vi "Actor Core.vi"(8 "error in":errorcluster, 11 "Arduino_Stepper in":refnum<class "Arduino_Stepper_UI.lvclass">) -> (0 "error out":errorcluster, 3 "Actor out":refnum<class "Actor.lvclass">)   [LabVIEW 2023, in "Arduino_TranslationStage_UI.lvlib" / "Arduino_Stepper_UI.lvclass"]
doc: "(<B>Filename</B>: Actor Framework.lvlib:Actor.lvclass:Actor Core.vi)\n\nReceives messages to the actor, reacts to them, and initiates any error handling that may shut the actor down.\n\nDescendant classes may override this VI to append parallel tasks for the actor to complete while it handles messages. Overrides use the Call Parent Class Method node."
uses:
  Arduino_Stepper_UI.lvclass
  C:/Program Files/National Instruments/LabVIEW 2023/vi.lib/ActorFramework/Actor/Actor.lvclass
  <vilib>/ActorFramework/Actor/Actor.lvclass
  <vilib>/ActorFramework/Message Enqueuer/Message Enqueuer.lvclass
  ConcreteClasses/ConcreteInstrumentClasses/Arduino_Stepper/Arduino_Stepper/ArduinoTranslationStage.lvclass
  <vilib>/ActorFramework/Actor/Actor.lvclass/Actor.ctl
  <vilib>/ActorFramework/Message Enqueuer/Message Enqueuer.lvclass/Message Enqueuer.ctl
  Arduino_Stepper_UI.lvclass/Arduino_Stepper_UI.ctl
  Top_Controllers/Spectroscopy_Controller/Camera_Scan_Controller Messages/Control_Init_Done Msg/Control_Init_Done Msg.lvclass/Control_Init_Done Msg.ctl
  Interfaces/InitDeinitInterface/InitDeinit Messages/Init Msg/Init Msg.lvclass/Init Msg.ctl
  Interfaces/AbstractInstrumentClasses/TranslationStages_LV/TranslationStagesInterface Messages/MoveBySteps Msg/MoveBySteps Msg.lvclass/MoveBySteps Msg.ctl
  Top_Controllers/Spectroscopy_Controller/Camera_Scan_Controller Messages/InitScan Msg/InitScan Msg.lvclass/InitScan Msg.ctl
  <vilib>/ActorFramework/Message Enqueuer/Init from Existing Queue.vi
  <vilib>/ActorFramework/Message Enqueuer/Enqueue.vi
  Top_Controllers/Spectroscopy_Controller/Camera_Scan_Controller Messages/Control_Init_Done Msg/Control_Init_Done Msg.lvclass
  C:/Program Files/National Instruments/LabVIEW 2023/vi.lib/ActorFramework/Message/Message.lvclass
  Interfaces/InitDeinitInterface/InitDeinit Messages/Init Msg/Init Msg.lvclass
  <vilib>/ActorFramework/Stop Msg/Stop Msg.lvclass
  Top_Controllers/Spectroscopy_Controller/Camera_Scan_Controller Messages/Control_DeInit_Done Msg/Control_DeInit_Done Msg.lvclass
  Interfaces/AbstractInstrumentClasses/TranslationStages_LV/TranslationStagesInterface Messages/MoveBySteps Msg/MoveBySteps Msg.lvclass
  Top_Controllers/Spectroscopy_Controller/Camera_Scan_Controller Messages/InitScan Msg/InitScan Msg.lvclass
  Top_Controllers/Spectroscopy_Controller/Camera_Scan_Controller Messages/Control_Moved Msg/Control_Moved Msg.lvclass
  <vilib>/ActorFramework/Message Priority Queue/Priority Enqueue.vi
panel:
  in  "Delay (ms)":u16(slide) max=5000 step=100 scale=0.0..5000.0
  out "Front Panel":refnum<vi>
  out "Is Top Actor":bool
  out "Caller Enqueuer":refnum<class "Message Enqueuer.lvclass">
  out "Direction":enum16{"Forward", "Backwards"}(ring)
  out "Scanning":bool=TRUE
  out "Moving":bool=TRUE
  out "Exited":bool=TRUE
  out "Connected":bool=TRUE
  out "Self Enqueuer":refnum<class "Message Enqueuer.lvclass">
  out "Arduino Enqueuer":refnum<class "Message Enqueuer.lvclass">
  out "VI":refnum<vi>
  in  "Get Images":bool
  in  "Scan Backwards":bool
  in  "Scan Forward":bool
  in  "Connect":bool
  in  "VISA resource name":refnum<visa-resource-name>
  in  "Jog Backwards":bool
  in  "Jog Forward":bool
  in  "Segments":dbl(slide) min=0.0 max=1000.0 step=1.0 scale=0.0..1000.0
  in  "Speed":dbl(slide)=100.0 min=100.0 max=2000.0 step=1.0 scale=100.0..2000.0
  in  "Steps":dbl(slide)=1.0 min=1.0 max=100000.0 step=1.0 scale=1.0..100000.0
  in  "Stop Button":bool
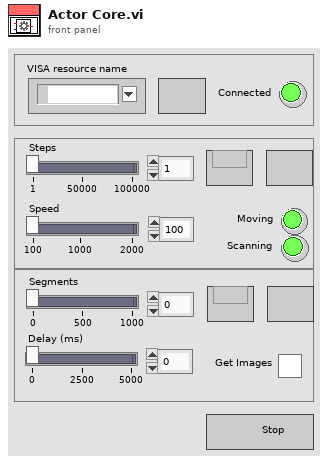
[diagram p1: front panel]
types:
  T1 = enum8{"Enabled", "Disabled", "Disabled and Grayed Out"}
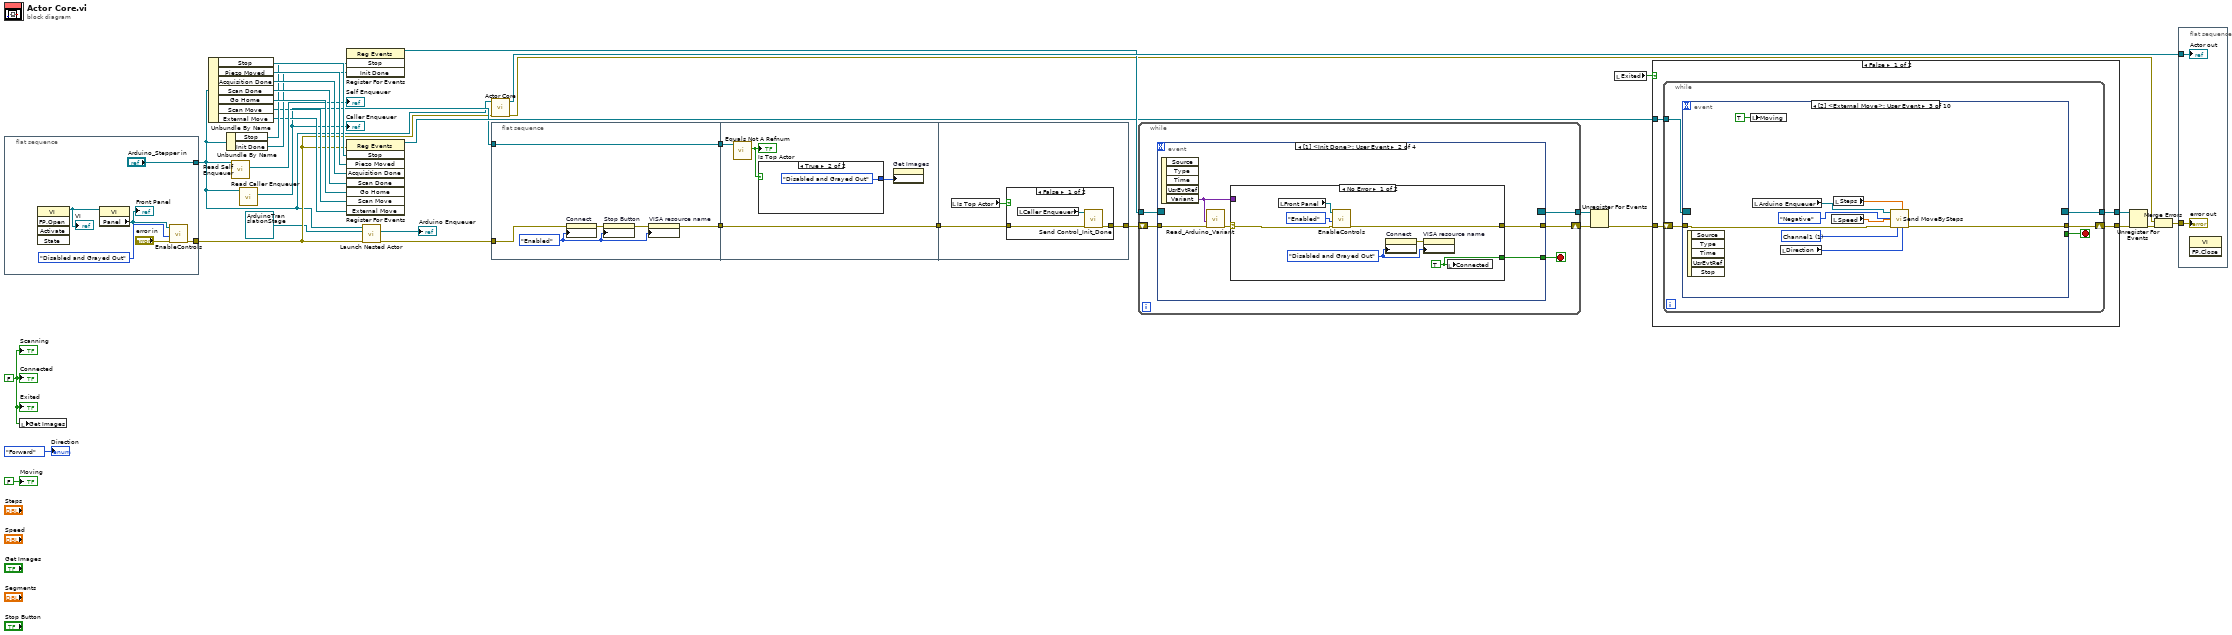
[diagram p0: block diagram]
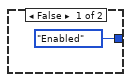
[diagram p2: hidden frame]
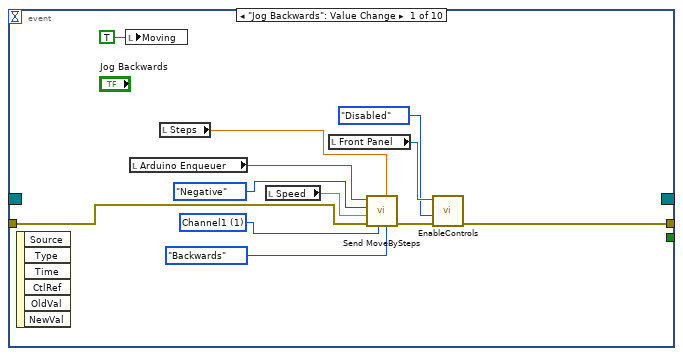
[diagram p4: hidden frame]
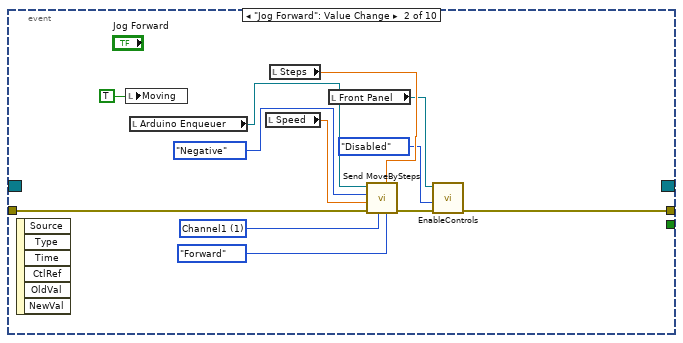
[diagram p5: hidden frame]
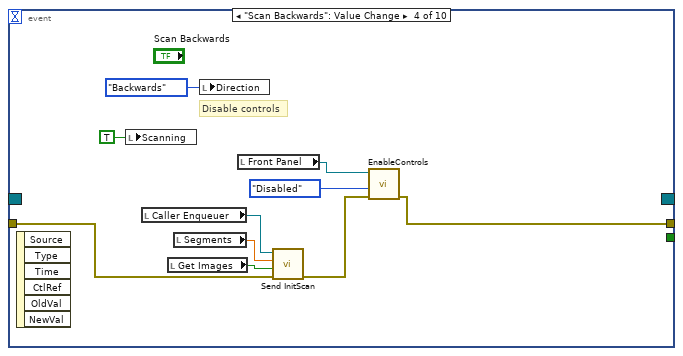
[diagram p6: hidden frame]
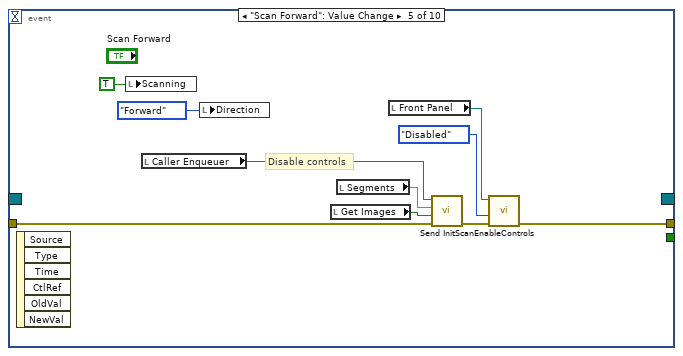
[diagram p7: hidden frame]
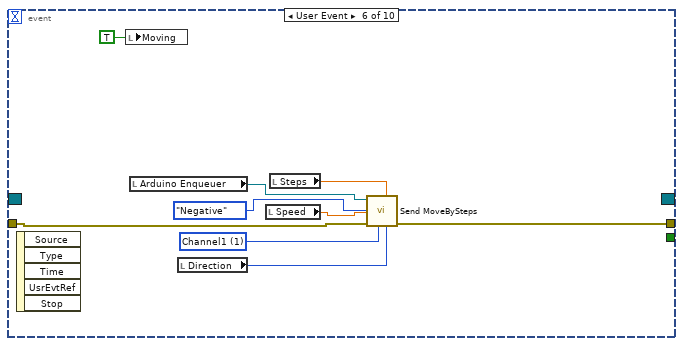
[diagram p8: hidden frame]
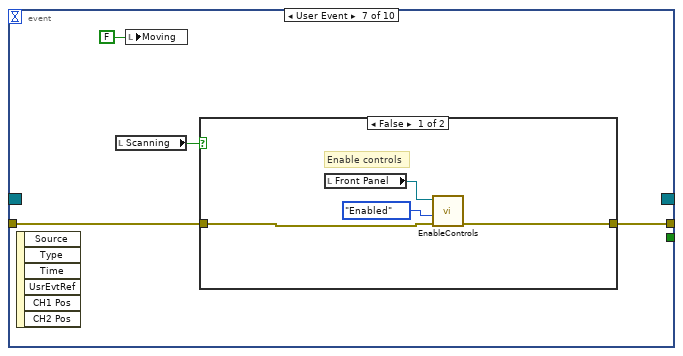
[diagram p9: hidden frame]
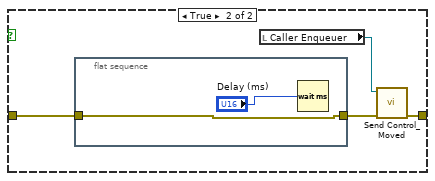
[diagram p10: hidden frame]
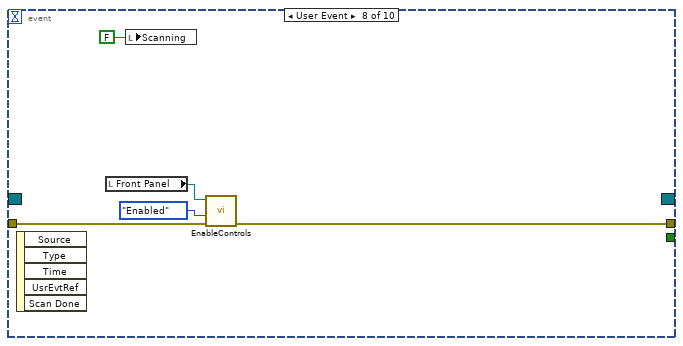
[diagram p11: hidden frame]
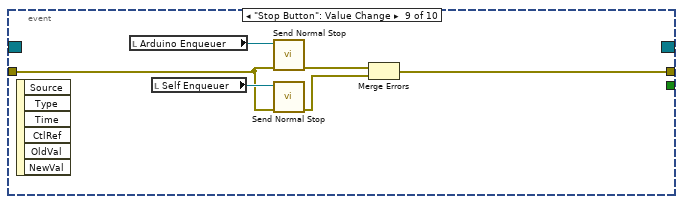
[diagram p12: hidden frame]
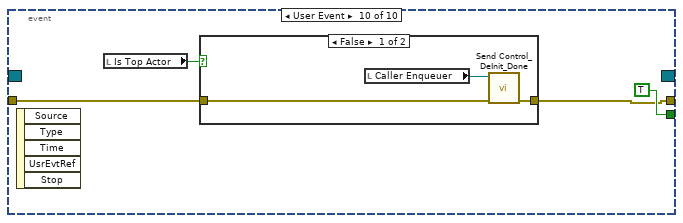
[diagram p13: hidden frame]
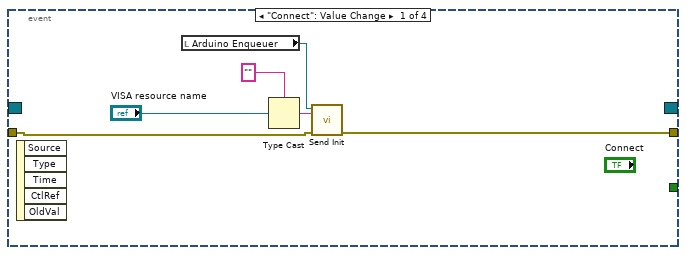
[diagram p16: hidden frame]
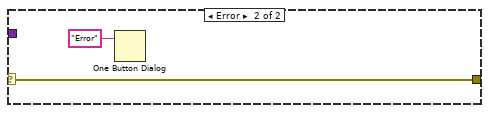
[diagram p17: hidden frame]
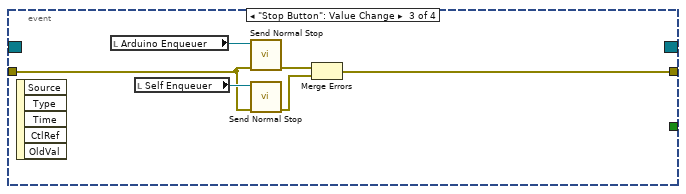
[diagram p18: hidden frame]
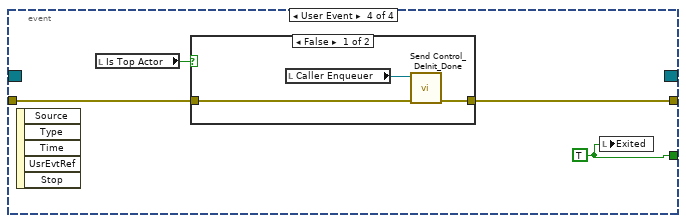
[diagram p19: hidden frame]
diagram:
  w1 = FALSE ("Capturing")
  n1 = flat-sequence {
    tunnel: ["Arduino_Stepper in"] -> w5
    tunnel: [w39] -> w6
    frame #0 {
      n2 = invoke class="VI" method="FP.Open"() -> (reference out=w37:refnum<vi>)  [unwired: 5 in, 4 out]
      "VI" <- w37
      n3 = property class="VI"(reference=w37) -> ("Panel"=w36:refnum<vi>)  [unwired: 1 in, 2 out]
      "Front Panel" <- w36
      n4 = call "EnableControls.vi"("error in (no error)"="error in", "Disabled"=T1."Disabled and Grayed Out", "Panel in"=w36) -> ("error out"=w39:errorcluster)  [unwired: 8 in]
    }
  }
  n5 = local write "Get Images"(w1) -> ()
  n6 = Unbundle By Name(w5) -> ("Stop"=w34:refnum<user-event>, "Piezo Moved"=w33:refnum<user-event>, "Acquisition Done"=w32:refnum<user-event>, "Scan Done"=w31:refnum<user-event>, "Go Home"=w30:refnum<user-event>, "Scan Move"=w14:refnum<user-event>, "External Move"=w11:refnum<user-event>)
  n7 = Unbundle By Name(w5) -> ("Stop"=w29:refnum<user-event>, "Init Done"=w28:refnum<user-event>)
  n8 = call <vilib>:"Read Self Enqueuer.vi"("Actor"=w5) -> ("Self Enqueuer"=→"Self Enqueuer":refnum<class "Message Enqueuer.lvclass">)  [unwired: 10 in]
  n9 = call <vilib>:"Read Caller Enqueuer.vi"("Actor"=w5) -> ("Caller Enqueuer"=w9:refnum<class "Message Enqueuer.lvclass">)  [unwired: 10 in]
  "Caller Enqueuer" <- w9
  n10 = register-events(w29, w28) -> (reference out=w27:refnum<event-registration>)  [unwired: 2 in, 1 out]
  n11 = register-events(error in=w6, w34, w33, w32, w31, w30, w14, w11) -> (reference out=w24:refnum<event-registration>)  [unwired: 1 in, 1 out]
  n12 = call <vilib>:"Launch Nested Actor.vi"("error in (no error)"=w6, "Nested Actor"=refnum<class "ArduinoTranslationStage.lvclass"> refnum ("ArduinoTranslationStage.lvlib:ArduinoTranslationStage.lvclass"), "Caller Actor in"=w5) -> ("error out"=w2:errorcluster, "Nested Actor's Enqueuer"=→"Arduino Enqueuer":refnum<class "Message Enqueuer.lvclass">)  [unwired: 6 in, 1 out]
  n13 = call-parent "Actor Core.vi"("error in"=w6, "Actor in"=w5) -> ("error out"=w19:errorcluster, "Actor out"=w35:refnum<class "Actor.lvclass">)  [unwired: 8 in]
  n14 = flat-sequence {
    tunnel: w9 -> [w47]
    tunnel: [w45] -> w8
    tunnel: [w47] -> w7
    tunnel: w2 -> [w46]
    tunnel: [w51] -> w10
    tunnel: w8 -> [w51]
    tunnel: w7 -> [w50]
    tunnel: [w54] -> w12
    tunnel: w10 -> [w55]
    frame #0 {
      w42 = T1."Enabled" ("Disabled")
      n15 = property on="Connect" class="Bool"(error in=w46, "DisabledEnum"=w42) -> (error out=w44:errorcluster)  [unwired: 1 in, 1 out]
      n16 = property on="Stop Button" class="Bool"(error in=w44, "DisabledEnum"=w42) -> (error out=w43:errorcluster)  [unwired: 1 in, 1 out]
      n17 = property on="VISA resource name" class="VISAName"(error in=w43, "DisabledEnum"=w42) -> (error out=w45:errorcluster)  [unwired: 1 in, 1 out]
    }
    frame #1 {
      n18 = call <vilib>:"Equals Not A Refnum.vi"("Message Enqueuer"=w50) -> ("Not a refnum?"=w49:bool)  [unwired: 10 in]
      "Is Top Actor" <- w49
      n19 = case shown="True" w49 {
        tunnel: [T1."Enabled" ("Disabled") T1."Disabled and Grayed Out" ("Disabled")] -> w48
        frame False {
        }
        frame True {
        }
      }
      n20 = property on="Get Images" class="Bool (strict)"("DisabledEnum"=w48) -> ()  [unwired: 2 in, 2 out]
    }
    frame #2 {
      n21 = local read "Is Top Actor"() -> (w56:bool)
      n22 = case shown="False" w56 {
        tunnel: w55 -> [w59 w60]
        tunnel: [w58 w60] -> w54
        frame False {
          n23 = local read "Caller Enqueuer"() -> (w57:refnum<class "Message Enqueuer.lvclass">)
          n24 = call "Send Control_Init_Done.vi"("error in (no error)"=w59, "Message Enqueuer"=w57) -> ("error out"=w58:errorcluster)  [unwired: 8 in, 1 out]
        }
        frame True {
        }
      }
    }
  }
  n25 = while {
    tunnel: w27 -> [w64]
    shift-right: [w63] -> w21
    shift-left: w12 -> [w65]
    tunnel: [w61] -> w22
    stop <- w62 stop-if-true
    n26 = event shown="[1] <Init Done>: User Event" {
      selector: w64 -> [_ _ _ _]
      dyn-events: [_ _ _ _] -> w61
      timeout: _ -> [_ _ _ _]
      tunnel: w65 -> [w67 w75 w89 w93]
      tunnel: [w66 w76 w86 w92] -> w63
      tunnel: [_ w73 _ w95] -> w62
      event "Connect": Value Change {
        n27 = event-data() -> ()  [unwired: 1 in, 5 out]
        n28 = local read "Arduino Enqueuer"() -> (w71:refnum<class "Message Enqueuer.lvclass">)
        n29 = Type Cast(type="" ("Address"), x="VISA resource name") -> (*(type *) &x=w70:string)
        n30 = call "Send Init.vi"("error in (no error)"=w67, "Address"=w70, "Message Enqueuer"=w71) -> ("error out"=w66:errorcluster)  [unwired: 7 in, 1 out]
      }
      event User Event {
        n31 = event-data() -> ("Variant"=w72:variant)  [unwired: 1 in, 4 out]
        n32 = call "Read_Arduino_Variant.vi"("error in (no error)"=w75, "Variant"=w72) -> ("error out"=w74:errorcluster)  [unwired: 8 in, 1 out]
        n33 = case shown="No Error" w74 {
          selector: w74 -> [w80 w84]
          tunnel: [w77 w84] -> w76
          tunnel: [w83 _] -> w73
          tunnel: w72 -> [_ _]
          frame No Error {
            w78 = T1."Disabled and Grayed Out" ("Disabled")
            w83 = TRUE
            n34 = local read "Front Panel"() -> (w81:refnum<vi>)
            n35 = call "EnableControls.vi"("error in (no error)"=w80, "Disabled"=T1."Enabled", "Panel in"=w81) -> ("error out"=w77:errorcluster)  [unwired: 8 in]
            n36 = property on="Connect" class="Bool"("DisabledEnum"=w78) -> (error out=w79:errorcluster)  [unwired: 2 in, 1 out]
            n37 = property on="VISA resource name" class="VISAName"(error in=w79, "DisabledEnum"=w78) -> ()  [unwired: 1 in, 2 out]
            n38 = local write "Connected"(w83) -> ()
          }
          frame Error {
            n39 = One Button Dialog(message="Error") -> ()  [unwired: 1 in, 1 out]
          }
        }
      }
      event "Stop Button": Value Change {
        n40 = event-data() -> ()  [unwired: 1 in, 5 out]
        n41 = local read "Arduino Enqueuer"() -> (w91:refnum<class "Message Enqueuer.lvclass">)
        n42 = local read "Self Enqueuer"() -> (w90:refnum<class "Message Enqueuer.lvclass">)
        n43 = call <vilib>:"Send Normal Stop.vi"("error in (no error)"=w89, "Message Enqueuer"=w91) -> ("error out"=w88:errorcluster)  [unwired: 9 in]
        n44 = call <vilib>:"Send Normal Stop.vi"("error in (no error)"=w89, "Message Enqueuer"=w90) -> ("error out"=w87:errorcluster)  [unwired: 9 in]
        n45 = Merge Errors(w88, w87) -> (w86:errorcluster)
      }
      event User Event {
        w95 = TRUE
        n46 = event-data() -> ()  [unwired: 1 in, 5 out]
        n47 = local read "Is Top Actor"() -> (w94:bool)
        n48 = case shown="False" w94 {
          tunnel: w93 -> [w97 w99]
          tunnel: [w96 w99] -> w92
          frame False {
            n49 = local read "Caller Enqueuer"() -> (w98:refnum<class "Message Enqueuer.lvclass">)
            n50 = call "Send Control_DeInit_Done.vi"("error in (no error)"=w97, "Message Enqueuer"=w98) -> ("error out"=w96:errorcluster)  [unwired: 8 in, 1 out]
          }
          frame True {
          }
        }
        n51 = local write "Exited"(w95) -> ()
      }
    }
  }
  n52 = Unregister For Events(event registration refnum=w22, error in=w21) -> (error out=w20:errorcluster)
  n53 = local read "Exited"() -> (w25:bool)
  n54 = case shown="False" w25 {
    tunnel: w20 -> [w103 w205]
    tunnel: [w102 w205] -> w17
    tunnel: w24 -> [w101 w204]
    tunnel: [w100 w204] -> w23
    frame False {
      n55 = while {
        shift-right: [w107] -> w102
        shift-left: w103 -> [w108]
        tunnel: w101 -> [w106]
        tunnel: [w105] -> w100
        stop <- w104 stop-if-true
        n56 = event shown="[2] <External Move>: User Event" {
          selector: w106 -> [_ _ _ _ _ _ _ _ _ _]
          dyn-events: [_ _ _ _ _ _ _ _ _ _] -> w105
          timeout: _ -> [_ _ _ _ _ _ _ _ _ _]
          tunnel: w108 -> [w114 w126 w135 w149 w159 w164 w171 w186 w190 w197]
          tunnel: [w109 w121 w137 w142 w152 w166 w172 w185 w191 w196] -> w107
          tunnel: [_ _ _ _ _ _ _ _ _ TRUE] -> w104
          event "Jog Backwards": Value Change {
            w116 = u16 1 items=["Channel1"=1, "Channel2"=2, "Channel3"=3, "Channel4"=4] ("Channel")
            n57 = event-data() -> ()  [unwired: 1 in, 6 out]
            n58 = local write "Moving"(TRUE ("Moving")) -> ()
            n59 = local read "Arduino Enqueuer"() -> (w120:refnum<class "Message Enqueuer.lvclass">)
            n60 = local read "Steps"() -> (w118:dbl)
            n61 = local read "Speed"() -> (w117:dbl)
            n62 = local read "Front Panel"() -> (w112:refnum<vi>)
            n63 = call "Send MoveBySteps.vi"("Direction"=enum16{"Forward", "Backwards"}."Backwards", "Steps"=w118, "Channel"=w116, "error in (no error)"=w114, "Speed"=w117, "Polarity"=enum16{"Positive", "Negative"}."Negative", "Message Enqueuer"=w120) -> ("error out"=w110:errorcluster)  [unwired: 3 in, 1 out]
            n64 = call "EnableControls.vi"("error in (no error)"=w110, "Disabled"=T1."Disabled", "Panel in"=w112) -> ("error out"=w109:errorcluster)  [unwired: 8 in]
          }
          event "Jog Forward": Value Change {
            w129 = u16 1 items=["Channel1"=1, "Channel2"=2, "Channel3"=3, "Channel4"=4] ("Channel")
            n65 = event-data() -> ()  [unwired: 1 in, 6 out]
            n66 = local write "Moving"(TRUE ("Moving")) -> ()
            n67 = local read "Arduino Enqueuer"() -> (w132:refnum<class "Message Enqueuer.lvclass">)
            n68 = local read "Speed"() -> (w131:dbl)
            n69 = local read "Steps"() -> (w127:dbl)
            n70 = local read "Front Panel"() -> (w124:refnum<vi>)
            n71 = call "Send MoveBySteps.vi"("Direction"=enum16{"Forward", "Backwards"}."Forward", "Steps"=w127, "Channel"=w129, "error in (no error)"=w126, "Speed"=w131, "Polarity"=enum16{"Positive", "Negative"}."Negative", "Message Enqueuer"=w132) -> ("error out"=w122:errorcluster)  [unwired: 3 in, 1 out]
            n72 = call "EnableControls.vi"("error in (no error)"=w122, "Disabled"=T1."Disabled", "Panel in"=w124) -> ("error out"=w121:errorcluster)  [unwired: 8 in]
          }
          event User Event {
            w139 = u16 1 items=["Channel1"=1, "Channel2"=2, "Channel3"=3, "Channel4"=4] ("Channel")
            n73 = event-data() -> ()  [unwired: 1 in, 5 out]
            n74 = local write "Moving"(TRUE ("Moving")) -> ()
            n75 = local read "Arduino Enqueuer"() -> (w141:refnum<class "Message Enqueuer.lvclass">)
            n76 = local read "Direction"() -> (w133:enum16{"Forward", "Backwards"})
            n77 = local read "Speed"() -> (w140:dbl)
            n78 = local read "Steps"() -> (w136:dbl)
            n79 = call "Send MoveBySteps.vi"("Direction"=w133, "Steps"=w136, "Channel"=w139, "error in (no error)"=w135, "Speed"=w140, "Polarity"=enum16{"Positive", "Negative"}."Negative", "Message Enqueuer"=w141) -> ("error out"=w137:errorcluster)  [unwired: 3 in, 1 out]
          }
          event "Scan Backwards": Value Change {
            # "Disable controls"
            n80 = event-data() -> ()  [unwired: 1 in, 6 out]
            n81 = local write "Scanning"(TRUE ("Scanning")) -> ()
            n82 = local read "Caller Enqueuer"() -> (w146:refnum<class "Message Enqueuer.lvclass">)
            n83 = local read "Get Images"() -> (w150:bool)
            n84 = local read "Segments"() -> (w151:dbl)
            n85 = local write "Direction"(enum16{"Forward", "Backwards"}."Backwards" ("Direction")) -> ()
            n86 = local read "Front Panel"() -> (w145:refnum<vi>)
            n87 = call "Send InitScan.vi"("error in (no error)"=w149, "Save Images?"=w150, "Total Steps"=w151, "Message Enqueuer"=w146) -> ("error out"=w143:errorcluster)  [unwired: 6 in, 1 out]
            n88 = call "EnableControls.vi"("error in (no error)"=w143, "Disabled"=T1."Disabled", "Panel in"=w145) -> ("error out"=w142:errorcluster)  [unwired: 8 in]
          }
          event "Scan Forward": Value Change {
            # "Disable controls"
            n89 = event-data() -> ()  [unwired: 1 in, 6 out]
            n90 = local write "Scanning"(TRUE ("Scanning")) -> ()
            n91 = local read "Caller Enqueuer"() -> (w156:refnum<class "Message Enqueuer.lvclass">)
            n92 = local write "Direction"(enum16{"Forward", "Backwards"}."Forward" ("Direction")) -> ()
            n93 = local read "Get Images"() -> (w160:bool)
            n94 = local read "Segments"() -> (w161:dbl)
            n95 = local read "Front Panel"() -> (w155:refnum<vi>)
            n96 = call "Send InitScan.vi"("error in (no error)"=w159, "Save Images?"=w160, "Total Steps"=w161, "Message Enqueuer"=w156) -> ("error out"=w153:errorcluster)  [unwired: 6 in, 1 out]
            n97 = call "EnableControls.vi"("error in (no error)"=w153, "Disabled"=T1."Disabled", "Panel in"=w155) -> ("error out"=w152:errorcluster)  [unwired: 8 in]
          }
          event User Event {
            w168 = u16 1 items=["Channel1"=1, "Channel2"=2, "Channel3"=3, "Channel4"=4] ("Channel")
            n98 = event-data() -> ()  [unwired: 1 in, 5 out]
            n99 = local write "Moving"(TRUE ("Moving")) -> ()
            n100 = local read "Arduino Enqueuer"() -> (w170:refnum<class "Message Enqueuer.lvclass">)
            n101 = local read "Direction"() -> (w162:enum16{"Forward", "Backwards"})
            n102 = local read "Speed"() -> (w169:dbl)
            n103 = local read "Steps"() -> (w165:dbl)
            n104 = call "Send MoveBySteps.vi"("Direction"=w162, "Steps"=w165, "Channel"=w168, "error in (no error)"=w164, "Speed"=w169, "Polarity"=enum16{"Positive", "Negative"}."Negative", "Message Enqueuer"=w170) -> ("error out"=w166:errorcluster)  [unwired: 3 in, 1 out]
          }
          event User Event {
            n105 = event-data() -> ()  [unwired: 1 in, 6 out]
            n106 = local read "Scanning"() -> (w173:bool)
            n107 = local write "Moving"(FALSE ("Moving")) -> ()
            n108 = case shown="False" w173 {
              tunnel: [w175 w182] -> w172
              tunnel: w171 -> [w176 w180]
              frame False {
                # "Enable controls"
                n109 = local read "Front Panel"() -> (w177:refnum<vi>)
                n110 = call "EnableControls.vi"("error in (no error)"=w176, "Disabled"=T1."Enabled", "Panel in"=w177) -> ("error out"=w175:errorcluster)  [unwired: 8 in]
              }
              frame True {
                n111 = flat-sequence {
                  tunnel: [w183] -> w179
                  tunnel: w180 -> [w183]
                  frame #0 {
                    n112 = Wait (ms)(milliseconds to wait="Delay (ms)") -> ()  [unwired: 1 out]
                  }
                }
                n113 = local read "Caller Enqueuer"() -> (w181:refnum<class "Message Enqueuer.lvclass">)
                n114 = call "Send Control_Moved.vi"("error in (no error)"=w179, "Message Enqueuer"=w181) -> ("error out"=w182:errorcluster)  [unwired: 8 in, 1 out]
              }
            }
          }
          event User Event {
            n115 = event-data() -> ()  [unwired: 1 in, 5 out]
            n116 = local read "Front Panel"() -> (w188:refnum<vi>)
            n117 = local write "Scanning"(FALSE ("Scanning")) -> ()
            n118 = call "EnableControls.vi"("error in (no error)"=w186, "Disabled"=T1."Enabled", "Panel in"=w188) -> ("error out"=w185:errorcluster)  [unwired: 8 in]
          }
          event "Stop Button": Value Change {
            n119 = event-data() -> ()  [unwired: 1 in, 6 out]
            n120 = local read "Arduino Enqueuer"() -> (w192:refnum<class "Message Enqueuer.lvclass">)
            n121 = local read "Self Enqueuer"() -> (w193:refnum<class "Message Enqueuer.lvclass">)
            n122 = call <vilib>:"Send Normal Stop.vi"("error in (no error)"=w190, "Message Enqueuer"=w192) -> ("error out"=w194:errorcluster)  [unwired: 9 in]
            n123 = call <vilib>:"Send Normal Stop.vi"("error in (no error)"=w190, "Message Enqueuer"=w193) -> ("error out"=w195:errorcluster)  [unwired: 9 in]
            n124 = Merge Errors(w194, w195) -> (w191:errorcluster)
          }
          event User Event {
            n125 = event-data() -> ()  [unwired: 1 in, 5 out]
            n126 = local read "Is Top Actor"() -> (w198:bool)
            n127 = case shown="False" w198 {
              tunnel: w197 -> [w201 w203]
              tunnel: [w200 w203] -> w196
              frame False {
                n128 = local read "Caller Enqueuer"() -> (w202:refnum<class "Message Enqueuer.lvclass">)
                n129 = call "Send Control_DeInit_Done.vi"("error in (no error)"=w201, "Message Enqueuer"=w202) -> ("error out"=w200:errorcluster)  [unwired: 8 in, 1 out]
              }
              frame True {
              }
            }
          }
        }
      }
    }
    frame True {
    }
  }
  n130 = Unregister For Events(event registration refnum=w23, error in=w17) -> (error out=w18:errorcluster)
  n131 = Merge Errors(w19, w18) -> (w16:errorcluster)
  n132 = flat-sequence {
    tunnel: w16 -> [w207]
    tunnel: w35 -> [w206]
    frame #0 {
      n133 = invoke class="VI" method="FP.Close"() -> ()  [unwired: 3 in, 3 out]
      "error out" <- w207
      "Actor out" <- w206
    }
  }
  "Connected" <- w1
  "Exited" <- w1
  "Moving" <- FALSE ("Moving")
  "Scanning" <- w1
  "Direction" <- enum16{"Forward", "Backwards"}."Forward" ("Direction")
